vi "Find Settings File.vi"(8 "Error In":errorcluster) -> (0 "Error Out":errorcluster, 2 "Settings Filepath":path, 3 "Was settings file found?":bool)   [LabVIEW 2022 SP3]
doc: "This VI returns the filepath to the ini file that contains the tool setting(s)."
panel:
  out "Folder One Level Up":path
  out "INI Files (VI's folder)":string[](array[string])
  out "Current VI's Folder":path
  # "Development\nControls or indicators that are useful for development or testing, but which are not outputs of the VI."
  # "Input\nInputs to the VI"
  # "Output\nOutputs of the VI"
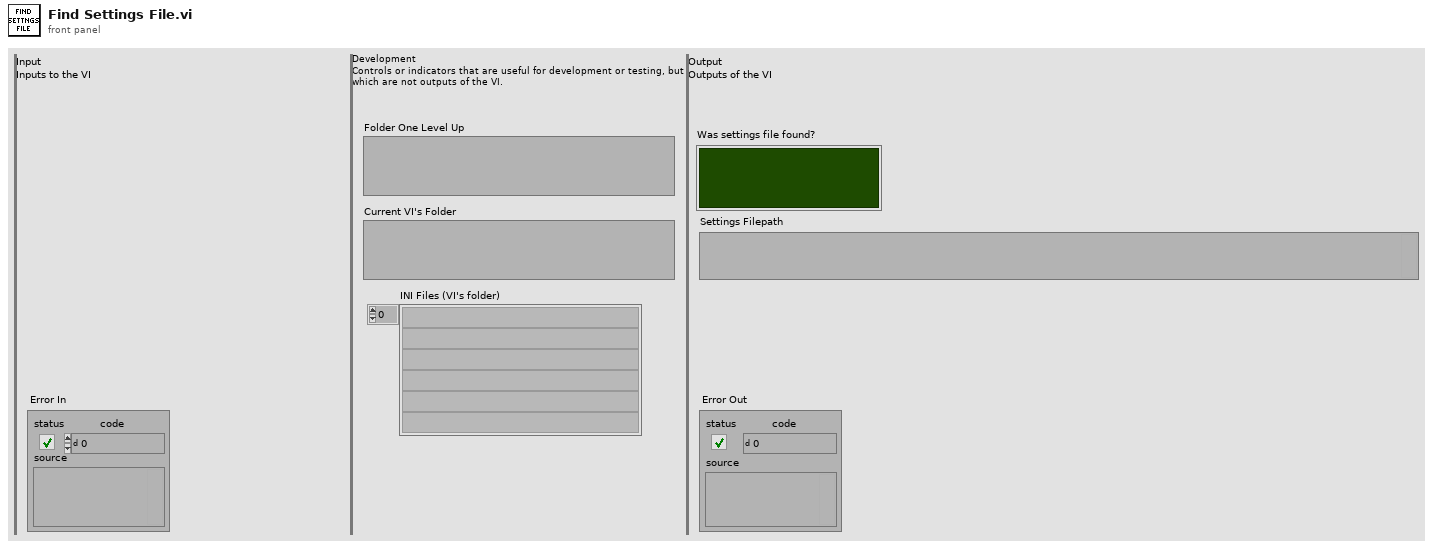
[diagram p1: front panel]
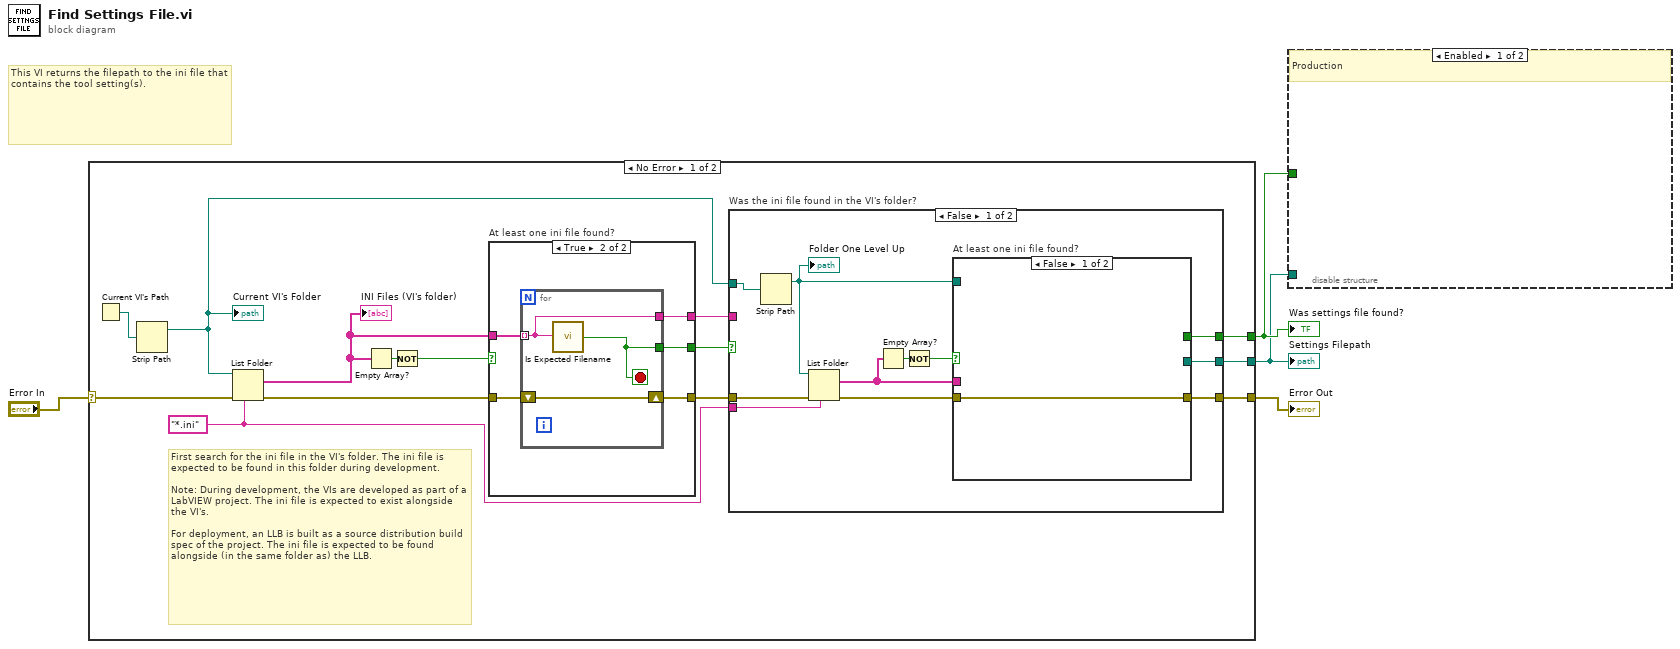
[diagram p0: block diagram]
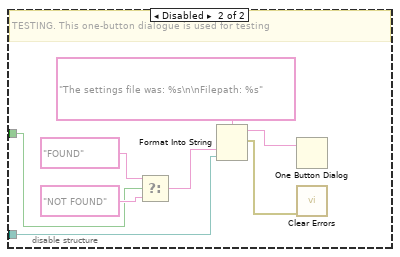
[diagram p2: hidden frame]
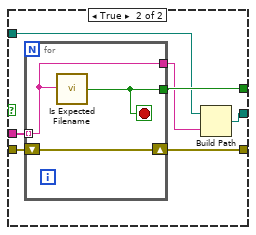
[diagram p4: hidden frame]
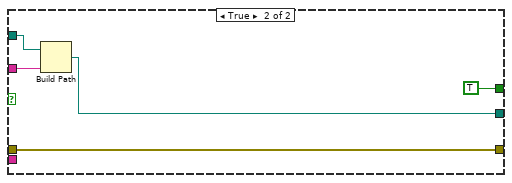
[diagram p5: hidden frame]
diagram:
  # "This VI returns the filepath to the ini file that contains the tool setting(s)."
  n1 = case shown="No Error" "Error In" {
    selector: "Error In" -> [w17 w55]
    tunnel: [w11 w55] -> w3
    tunnel: [w7 _] -> w2
    tunnel: [w5 _] -> w1
    frame No Error {
      w8 = "*.ini" ("pattern")
      # "First search for the ini file in the VI's folder. The ini file is expected to be found in this folder during development.\n\nNote: During development, the VIs are developed as part of a LabVIEW project. The ini file is expected to exist alongside the VI's.\n\nFor deployment, an LLB is built as a source distribution build spec of the project. The ini file is expected to be found alongside (in the same folder as) the LLB."
      n2 = Current VI's Path() -> (path=w18:path)
      n3 = Strip Path(path=w18) -> (stripped path=w9:path)  [unwired: 1 out]
      "Current VI's Folder" <- w9
      n4 = List Folder(path=w9, pattern=w8, error in=w17) -> (filenames=w12:string[], error out=w16:errorcluster)  [unwired: 1 in, 2 out]
      "INI Files (VI's folder)" <- w12
      n5 = Empty Array?(array=w12) -> (empty?=w14:bool)
      n6 = Not(x=w14) -> (.not. x?=w13:bool)
      n7 = case "At least one ini file found?" shown="True" w13 {
        tunnel: w16 -> [w19 w24]
        tunnel: [w19 w23] -> w15
        tunnel: w12 -> [_ w22]
        tunnel: [_ w21] -> w10
        tunnel: [_ w20] -> w6
        frame False {
        }
        frame True {
          n8 = for {
            shift-right: [w27] -> w23
            shift-left: w24 -> [w27]
            tunnel: w22 -> [w25] mode=indexing
            tunnel: [w26] -> w21
            tunnel: [w25] -> w20
            stop <- w26 stop-if-true
            n9 = call "Is Expected Filename.vi"("Filename"=w25) -> ("Matches the expected settings filename?"=w26:bool)
          }
        }
      }
      n10 = case "Was the ini file found in the VI's folder?" shown="False" w10 {
        tunnel: w15 -> [w37 w54]
        tunnel: [w34 w54] -> w11
        tunnel: w9 -> [w38 w53]
        tunnel: w8 -> [w36 _]
        tunnel: [w30 TRUE ("Matches the expected settings filename?")] -> w7
        tunnel: w6 -> [_ w52]
        tunnel: [w28 w51] -> w5
        frame False {
          n11 = Strip Path(path=w38) -> (stripped path=w29:path)  [unwired: 1 out]
          "Folder One Level Up" <- w29
          n12 = List Folder(path=w29, pattern=w36, error in=w37) -> (filenames=w32:string[], error out=w35:errorcluster)  [unwired: 1 in, 2 out]
          n13 = Empty Array?(array=w32) -> (empty?=w33:bool)
          n14 = Not(x=w33) -> (.not. x?=w31:bool)
          n15 = case "At least one ini file found?" shown="False" w31 {
            tunnel: w35 -> [w39 w46]
            tunnel: [w39 w45] -> w34
            tunnel: w32 -> [_ w44]
            tunnel: [_ w43] -> w30
            tunnel: w29 -> [_ w42]
            tunnel: [_ w40] -> w28
            frame False {
            }
            frame True {
              n16 = for {
                shift-right: [w49] -> w45
                shift-left: w46 -> [w49]
                tunnel: [w48] -> w43
                tunnel: w44 -> [w47] mode=indexing
                tunnel: [w47] -> w41
                stop <- w48 stop-if-true
                n17 = call "Is Expected Filename.vi"("Filename"=w47) -> ("Matches the expected settings filename?"=w48:bool)
              }
              n18 = Build Path(base path=w42, name or relative path=w41) -> (appended path=w40:path)
            }
          }
        }
        frame True {
          n19 = Build Path(base path=w53, name or relative path=w52) -> (appended path=w51:path)
        }
      }
    }
    frame Error {
    }
  }
  "Error Out" <- w3
  "Was settings file found?" <- w2
  "Settings Filepath" <- w1
  n20 = disable-structure shown="Enabled" {
    disable-tunnel: w2 -> [_ w61]
    disable-tunnel: w1 -> [_ w58]
    frame Enabled {
      # "Production"
    }
    frame Disabled {
      # "TESTING. This one-button dialogue is used for testing"
      n21 = Select(t="FOUND", s=w61, f="NOT FOUND") -> (s? t:f=w60:string)
      n22 = Format Into String(format string="The settings file was: %s\n\nFilepath: %s", w60, w58) -> (resulting string=w57:string, error out=w56:errorcluster)  [unwired: 2 in]
      n23 = One Button Dialog(message=w57) -> ()  [unwired: 1 in, 1 out]
      n24 = call <vilib>:"Clear Errors.vi"("error in (no error)"=w56) -> ()  [unwired: 5 in, 2 out]
    }
  }
